vi "Read Output Map.vi"(11 "OPC UA Client runtime in":refnum<class "OPC UA Client runtime.lvclass">) -> (2 "Output Map":T3(array[cluster]) {"OPC UA Data Type" items=["Boolean"=1, "SByte"=2, "Byte"=3, "Int16"=4, "UInt16"=5, "Int32"=6, "UInt32"=7, "Int64"=8, "UInt64"=9, "Float"=10, "Double"=11, "String"=12, "DateTime"=13, "ByteString"=15, "Array of Boolean"=101, "Array of SByte"=102, "Array of Byte"=103, "Array of Int16"=104, "Array of UInt16"=105, "Array of Int32"=106, "Array of UInt32"=107, "Array of Int64"=108, "Array of UInt64"=109, "Array of Float"=110, "Array of Double"=111, "Array of String"=112, "Array of DateTime"=113, "Array of ByteString"=115]}, 3 "OPC UA Client runtime out":refnum<class "OPC UA Client runtime.lvclass">)   [LabVIEW 2013, in "OPC UA Client runtime.lvclass"]
uses:
  OPC UA Client runtime.lvclass
  <vilib>/NI/Tag Bus/tag/Data Type.ctl
  configuration/OPC UA Data Type.ctl
  OPC UA Client runtime.lvclass/OPC UA Client runtime.ctl
  <vilib>/NI/Tag Bus/tag/tag descriptor.lvclass
  configuration/OPC UA Client configuration.lvclass
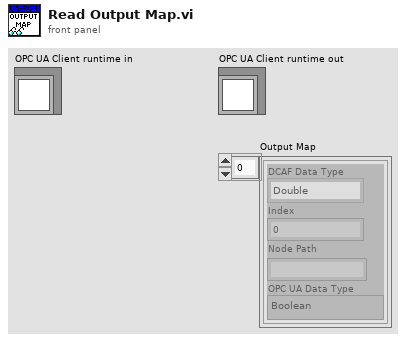
[diagram p1: front panel]
types:
  T1 = typedef "tag bus.lvlib/tag descriptor.lvclass/Data Type.ctl" = enum16{"Double", "Single", "I64", "I32", "I16", "I8", "U64", "U32", "U16", "U8", "Boolean", "String", "Array of Double", "Array of Single", "Array of I64", "Array of I32", "Array of I16", "Array of I8", "Array of U64", "Array of U32", "Array of U16", "Array of U8", "Array of Boolean", "Array of String"}
  T2 = typedef "OPC UA Client configuration.lvclass/OPC UA Data Type.ctl" = u16
  T3 = cluster{"DCAF Data Type":T1, "Index":i32, "Node Path":string, "OPC UA Data Type":T2}[]
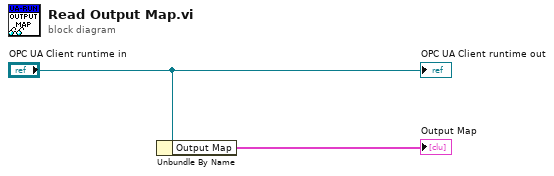
[diagram p0: block diagram]
diagram:
  n1 = Unbundle By Name("OPC UA Client runtime in") -> ("Output Map"=→"Output Map":T3)
  "OPC UA Client runtime out" <- "OPC UA Client runtime in"
